vi "Append Header, Footer and Watermark.vi"(6 "error in (no error)":errorcluster, 9 "PDF Report IN":T21(xcontrol)) -> (0 "error out":errorcluster, 2 "Path":path)   [LabVIEW 2013]
doc: "Location: at the end of the report generation.\n\nThis can only be followed by \"Print PDF.vi\" and \"Dispose references.vi\".\n\nVersion 1.0\nDeveloped by Jean-Marc Simard\nCopyright © 2010, Exaprom Inc.\nAll rights reserved.\nLicense: BSD\n\nWith iTextSharp Library\n(http://itextsharp.sourceforge.net)"
uses:
  Controls/PDF Report Xcontrol/PDF Report.xctl
  Controls/Page dimensions.ctl
  Controls/Page Orientation.ctl
  Controls/Header or Footer.ctl
  C:/Users/MaxCorp/Documents/GitHub/TopView/DLL/itextsharp.dll
  DLL/itextsharp.dll
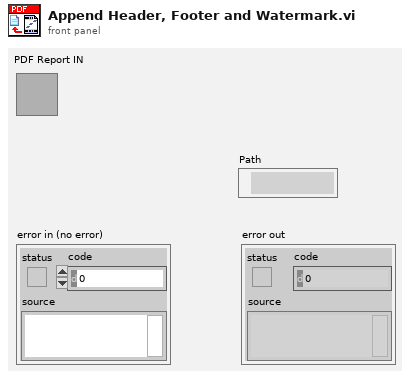
[diagram p1: front panel]
types:
  T1 = typedef "Font cluster.ctl" = cluster{"Name":string, "Size":T2, "Color":T3, "Style":cluster{"Bold":bool, "Italic":bool, "Underline":bool, "Strikeout":bool}}
  T2 = typedef "Font size.ctl" = sgl
  T3 = typedef "Font color.ctl" = u32
  T4 = typedef "Unit.ctl" = enum16{"inch", "mm"}
  T5 = typedef "Paragraphe cluster.ctl" = cluster{" Aligment":T6, "Line spacing":T7}
  T6 = typedef "Texte alignement.ctl" = enum16{"Select", "CENTER", "JUSTIFY", "LEFT", "RIGHT"}
  T7 = typedef "Line spacing.ctl" = enum16{"Select", "1.0", "1.5", "2.0"}
  T8 = typedef "Page dimensions.ctl" = cluster{"Start at page":i32, "Orientation":T9, "widht":sgl, "height":sgl, "Margin left":sgl, "Margin right":sgl, "Margin top":sgl, "Margin bottom":sgl}
  T9 = typedef "Page Orientation.ctl" = enum16{"Portrait", "Landscape"}
  T10 = typedef "Image or Table Caption.ctl" = cluster{"Caption":string, "Separator":string, "Position":enum16{"Above", "Below"}}
  T11 = typedef "Header Footer [ ].ctl" = T12[]
  T12 = typedef "Header Footer cluster.ctl" = cluster{"Start page":i32, "Type":T13, "Alignment":T14, "Vertical Alignement":T15, "Image (%)":sgl, "Page #":T16, "Text":string, "Path":string, "Font":T1, "Font refnum":refnum<k24>, "Line":cluster{"Line":T17, "Thickness (points)":sgl, "Colour":T3}}
  T13 = typedef "Header Footer Type.ctl" = enum16{"Select", "Text", "Text + hyperlink", "Page number", "Image", "Image + hyperlink"}
  T14 = typedef "Header footer horiz alignment.ctl" = enum16{"Left", "Center", "Right"}
  T15 = typedef "Cell Vertical alignment.ctl" = enum16{"TOP", "MIDDLE", "BOTTOM"}
  T16 = typedef "Page number.ctl" = cluster{"Text 1":string, "Text 2":string, "Text 3":string}
  T17 = typedef "Header Footer Line.ctl" = enum16{"No line", "Horizontal line"}
  T18 = typedef "Watermark cluster2.ctl" = cluster{"Show? (F)":bool, "Type":enum16{"Image", "Text"}, "Opacity (%)":sgl, "Rotate(°)":sgl, "Position":cluster{"Position":T19, "X":sgl, "Y":sgl}, "Image path":path, "Scaled(%)":sgl, "Image refnum":refnum<k24>, "Text":string, "Font":cluster{"Name":string, "Size":T2, "Color":T3}, "Font refnum":refnum<k24>, "Alignment":T14, "Automatic":bool}
  T19 = typedef "Watermark Position.ctl" = enum16{"Absolute", "Center (page)", "Center (text section)"}
  T20 = typedef "System Fonts.ctl" = cluster{"Font name [ ]":string[], "Font and file names [ ]":cluster{"Font name":string, "File name":string}[]}
  T21 = cluster{"Document":refnum<k24>, "Writer":refnum<k24>, "Default Font":refnum<k24>, "Default Font cluster":T1, "Path":path, "Unit (default = mm)":T4, "Paragraphe cluster":T5, "Pages dimensions [ ]":T8[], "Captions":cluster{"Image":T10, "Image counter":u16, "Table":T10, "Table counter":u16, "Font":T1}, "Header":T11, "Footer":T11, "Watermark ":T18, "Actual VI name":string, "System Fonts":T20}
  T22 = typedef "Header or Footer.ctl" = enum16{"Header", "Footer"}
  T23 = typedef "Header Footer Complete Cluster.ctl" = cluster{"Table position":cluster{"FixedHeight":dbl, "Table X postion":dbl, "Table Y postion":dbl}, "Header Footer Cluster with references [ ]":T24[]}
  T24 = typedef "Header Footer Cluster with references.ctl" = cluster{"Start page":i32, "Type":T13, "Alignment":T14, "Vertical Alignement":T15, "Page #":T16, "Text":refnum<k24>, "Scaled Img":refnum<k24>, "PdfPCell":refnum<k24>, "PdfPTable":refnum<k24>, "Font Cluster":T1, "Font ":refnum<k24>, "Img (%)":sgl, "Line":cluster{"Line":T17, "Thickness (points)":sgl, "Colour":T3}}
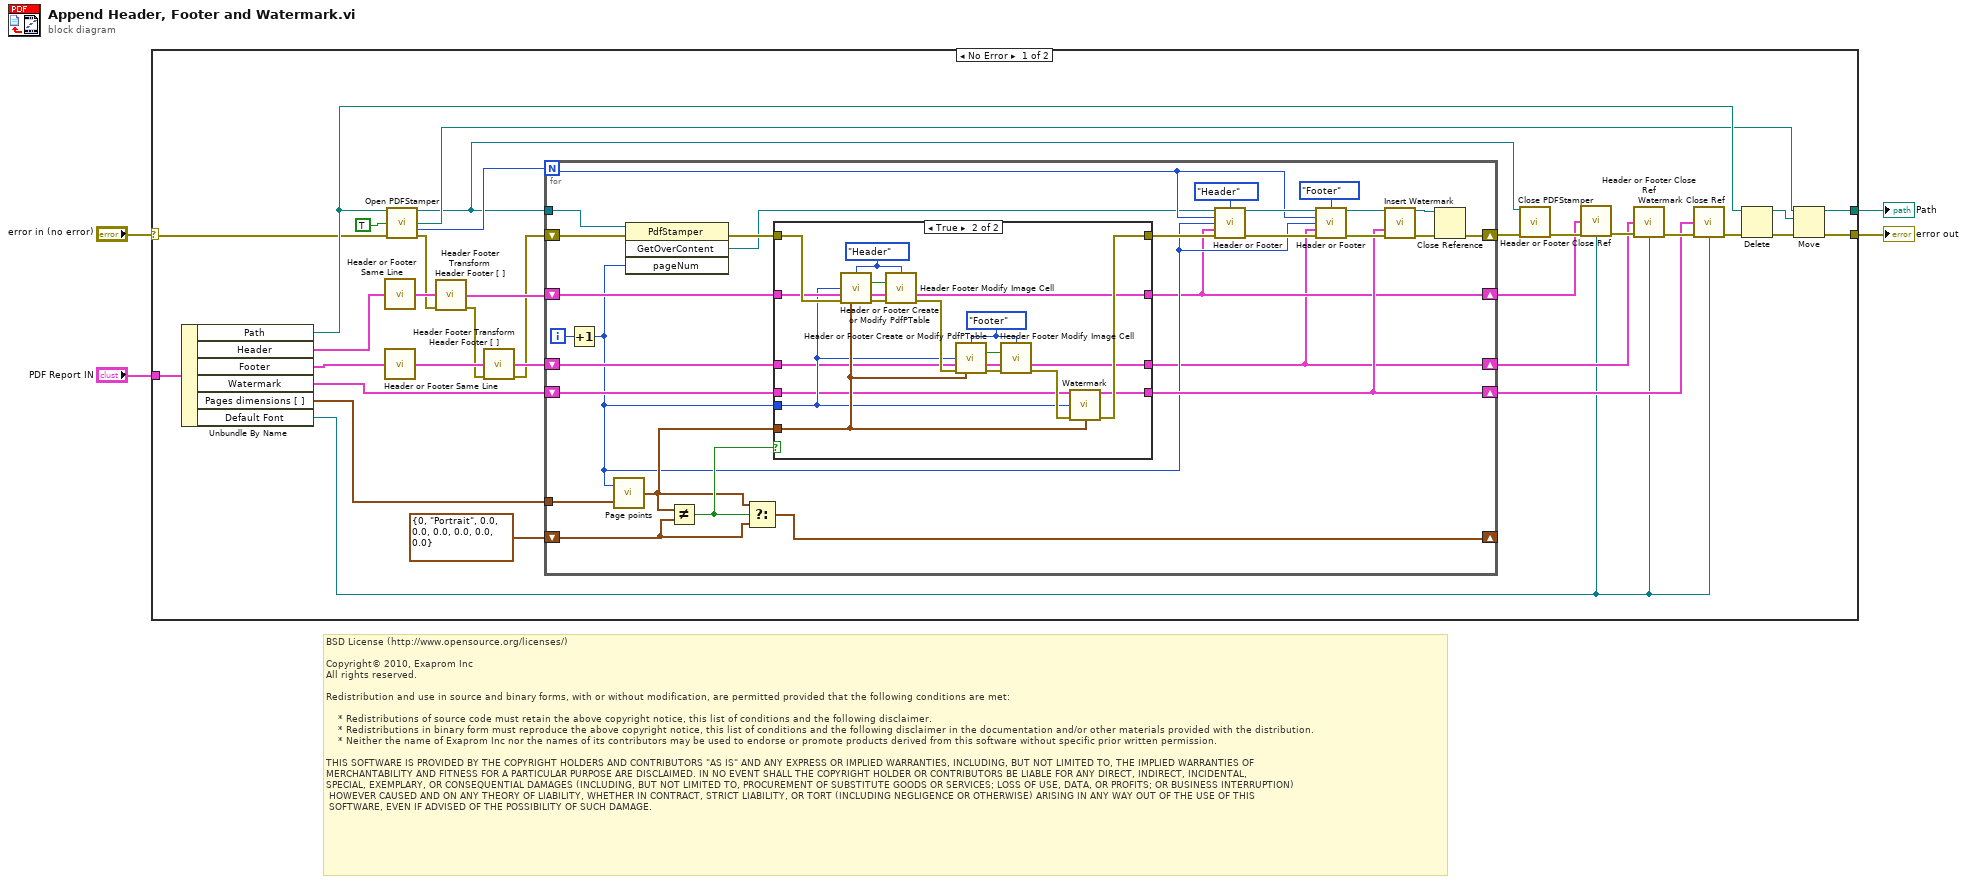
[diagram p0: block diagram]
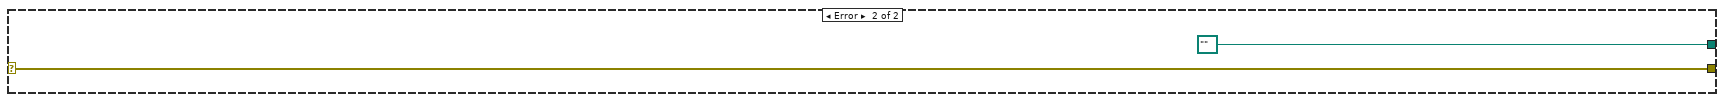
[diagram p3: hidden frame]
diagram:
  # "BSD License (http://www.opensource.org/licenses/)\n\nCopyright© 2010, Exaprom Inc\nAll rights reserved.\n\nRedistribution and use in source and binary forms, with or without modification, are permitted provided that the following conditions are met:\n\n    * Redistributions of source code must retain the above copyright notice, this list of conditions and the following disclaimer.\n    * Redistributions in binary form must reproduce the above copyright notice, this list of conditions and the following disclaimer in the documentation and/or other materials provided with the distribution.\n    * Neither the name of Exaprom Inc nor the names of its contributors may be used to endorse or promote products derived from this software without specific prior written permission.\n\nTHIS SOFTWARE IS PROVIDED BY THE COPYRIGHT HOLDERS AND CONTRIBUTORS \"AS IS\" AND ANY EXPRESS OR IMPLIED WARRANTIES, INCLUDING, BUT NOT LIMITED TO, THE IMPLIED WARRANTIES OF \nMERCHANTABILITY AND FITNESS FOR A PARTICULAR PURPOSE ARE DISCLAIMED. IN NO EVENT SHALL THE COPYRIGHT HOLDER OR CONTRIBUTORS BE LIABLE FOR ANY DIRECT, INDIRECT, INCIDENTAL,\nSPECIAL, EXEMPLARY, OR CONSEQUENTIAL DAMAGES (INCLUDING, BUT NOT LIMITED TO, PROCUREMENT OF SUBSTITUTE GOODS OR SERVICES; LOSS OF USE, DATA, OR PROFITS; OR BUSINESS INTERRUPTION)\n HOWEVER CAUSED AND ON ANY THEORY OF LIABILITY, WHETHER IN CONTRACT, STRICT LIABILITY, OR TORT (INCLUDING NEGLIGENCE OR OTHERWISE) ARISING IN ANY WAY OUT OF THE USE OF THIS\n SOFTWARE, EVEN IF ADVISED OF THE POSSIBILITY OF SUCH DAMAGE."
  n1 = case shown="No Error" "error in (no error)" {
    selector: "error in (no error)" -> [w34 w90]
    tunnel: [w5 w90] -> w4
    tunnel: "PDF Report IN" -> [w33 _]
    tunnel: [w35 path "" ("new path")] -> w1
    frame No Error {
      n2 = Unbundle By Name(w33) -> ("Path"=w36:path, "Header"=w31:T11, "Footer"=w32:T11, "Watermark"=w30:T18, "Pages dimensions [ ]"=w29:T8[], "Default Font"=w6:refnum<k24>)
      n3 = call "Header or Footer Same Line.vi"("Header Footer [ ] IN"=w31) -> ("Header Footer [ ] OUT"=w18:T11)
      n4 = call "Header or Footer Same Line.vi"("Header Footer [ ] IN"=w32) -> ("Header Footer [ ] OUT"=w16:T11)
      n5 = call "Open PDFStamper.vi"("PDF Path"=w36, "RotateContents (F)"=TRUE, "error in (no error)"=w34) -> ("PDFStamper"=w19:refnum<k24>, "Temporary File Name"=w25:path, "NumberOfPages"=w27:i32, "error out"=w13:errorcluster)  [unwired: 9 out]
      n6 = call "Header Footer Transform Header Footer [ ].vi"("Header or Footer [ ]"=w18, "error in (no error)"=w13) -> ("Header or Footer Complete Cluster"=w17:T23, "error out"=w14:errorcluster)  [unwired: 12 out]
      n7 = call "Header Footer Transform Header Footer [ ].vi"("Header or Footer [ ]"=w16, "error in (no error)"=w14) -> ("Header or Footer Complete Cluster"=w15:T23, "error out"=w12:errorcluster)  [unwired: 12 out]
      n8 = for {
        N: w27 -> [w52]
        tunnel: w19 -> [w58]
        tunnel: w29 -> [w53]
        shift-right: [w51] -> _
        shift-left: T8 {"Start at page"=0, "Orientation"=enum."Portrait", "widht"=0.0, "height"=0.0, "Margin left"=0.0, "Margin right"=0.0, "Margin top"=0.0, "Margin bottom"=0.0} ("Page (points)") -> [w50]
        shift-right: [w45] -> w7
        shift-left: w30 -> [w44]
        shift-right: [w43] -> w26
        shift-left: w12 -> [w59]
        shift-right: [w39] -> w11
        shift-left: w17 -> [w48]
        shift-right: [w38] -> w10
        shift-left: w15 -> [w46]
        i -> [w60]
        n9 = Increment(x=w60) -> (x+1=w40:i32)
        n10 = call "Page points.vi"("Pages dimensions [ ]"=w53, "pageNum"=w40) -> ("Page (points)"=w47:T8)
        n11 = invoke class="PdfStamper" method="GetOverContent"(reference=w58, error in=w59, "pageNum"=w40) -> (error out=w63:errorcluster, "GetOverContent"=w37:refnum<k24>)  [unwired: 1 in, 2 out]
        n12 = Not Equal?(x=w47, y=w50) -> (x != y?=w49:bool)
        n13 = Select(t=w47, s=w49, f=w50) -> (s? t:f=w51:T8)
        n14 = case shown="True" w49 {
          tunnel: w48 -> [w67 w84]
          tunnel: w47 -> [_ w80]
          tunnel: w46 -> [w66 w71]
          tunnel: w63 -> [w65 w88]
          tunnel: [w65 w86] -> w64
          tunnel: w44 -> [w68 w76]
          tunnel: [w68 w81] -> w45
          tunnel: w40 -> [_ w79]
          tunnel: [w67 w73] -> w39
          tunnel: [w66 w72] -> w38
          frame False {
          }
          frame True {
            w77 = Header_or_Footer."Footer" ("Header or Footer")
            w78 = Header_or_Footer."Header" ("Header or Footer")
            n15 = call "Header or Footer Create or Modify PdfPTable.vi"("Header or Footer"=w78, "pageNum"=w79, "Header Footer IN [ ]"=w84, "error in (no error)"=w88, "Page points"=w80) -> ("Modify Image Cell"=w70:bool, "Header Footer OUT [ ]"=w74:T23, "error out"=w83:errorcluster)  [unwired: 3 in, 5 out]
            n16 = call "Header Footer Modify Image Cell.vi"("Header or Footer"=w78, "Modify Image Cell"=w70, "Header or Footer Complete Cluster IN"=w74, "error in (no error)"=w83) -> ("Header or Footer Complete Cluster OUT"=w73:T23, "error out"=w85:errorcluster)  [unwired: 1 in, 9 out]
            n17 = call "Header or Footer Create or Modify PdfPTable.vi"("Header or Footer"=w77, "pageNum"=w79, "Header Footer IN [ ]"=w71, "error in (no error)"=w85, "Page points"=w80) -> ("Modify Image Cell"=w69:bool, "Header Footer OUT [ ]"=w75:T23, "error out"=w82:errorcluster)  [unwired: 3 in, 5 out]
            n18 = call "Header Footer Modify Image Cell.vi"("Header or Footer"=w77, "Modify Image Cell"=w69, "Header or Footer Complete Cluster IN"=w75, "error in (no error)"=w82) -> ("Header or Footer Complete Cluster OUT"=w72:T23, "error out"=w87:errorcluster)  [unwired: 1 in, 9 out]
            n19 = call "Watermark.vi"("Watermark IN"=w76, "pageNum"=w79, "error in (no error)"=w87, "Page dimensions"=w80) -> ("Watermark OUT"=w81:T18, "error out"=w86:errorcluster)  [unwired: 2 in, 8 out]
          }
        }
        n20 = call "Header or Footer.vi"("OverContent"=w37, "Header or Footer"=Header_or_Footer."Header", "NumberOfPages"=w52, "pageNum"=w40, "Header or Footer Complete Cluster"=w39, "error in (no error)"=w64) -> ("OverContent duplicate"=w61:refnum<k24>, "error out"=w62:errorcluster)  [unwired: 2 in, 6 out]
        n21 = call "Header or Footer.vi"("OverContent"=w61, "Header or Footer"=Header_or_Footer."Footer", "NumberOfPages"=w52, "pageNum"=w40, "Header or Footer Complete Cluster"=w38, "error in (no error)"=w62) -> ("OverContent duplicate"=w56:refnum<k24>, "error out"=w57:errorcluster)  [unwired: 1 in, 7 out]
        n22 = call "Insert Watermark.vi"("OverContent"=w56, "Watermark Cluster"=w45, "error in (no error)"=w57) -> ("OverContent duplicate"=w54:refnum<k24>, "error out"=w55:errorcluster)  [unwired: 3 in, 8 out]
        n23 = Close Reference(reference=w54, error in (no error)=w55) -> (error out=w43:errorcluster)
      }
      n24 = call "Close PDFStamper.vi"("PDFStamper"=w19, "error in (no error)"=w26) -> ("error out"=w21:errorcluster)  [unwired: 13 out]
      n25 = call "Header or Footer Close Ref.vi"("Header or Footer Complete Cluster"=w11, "error in (no error)"=w21, "Default Font"=w6) -> ("error out"=w20:errorcluster)  [unwired: 1 in, 11 out]
      n26 = call "Header or Footer Close Ref.vi"("Header or Footer Complete Cluster"=w10, "error in (no error)"=w20, "Default Font"=w6) -> ("error out"=w9:errorcluster)  [unwired: 12 out]
      n27 = call "Watermark Close Ref.vi"("Watermark IN"=w7, "error in (no error)"=w9, "Default Font"=w6) -> ("error out"=w8:errorcluster)  [unwired: 12 out]
      n28 = Delete(path (use dialog)=w36, error in=w8) -> (deleted path=w23:path, error out=w22:errorcluster)  [unwired: 4 out]
      n29 = Move(source path=w25, error in=w22, 10:w23) -> (error out=w5:errorcluster, 3:w35:path)  [unwired: 3 out]
    }
    frame Error {
    }
  }
  "error out" <- w4
  "Path" <- w1
